vi "Process buy UI.vi"(8 "error in (no error)":errorcluster, 11 "UI Actor in":refnum<class "UI Actor.lvclass">) -> (0 "error out":errorcluster, 3 "UI Actor out":refnum<class "UI Actor.lvclass">)   [LabVIEW 2020, in "UI Actor.lvlib" / "UI Actor.lvclass"]
uses:
  UI Actor.lvclass
  C:/Program Files/National Instruments/LabVIEW 2020/vi.lib/ActorFramework/Actor/Actor.lvclass
  UI Actor.lvclass/UI Actor.ctl
  coffe actor Messages/Productos inventario coffee Msg/Productos inventario coffee Msg.lvclass/Productos inventario coffee Msg.ctl
  <vilib>/ActorFramework/Message Enqueuer/Message Enqueuer.lvclass/Message Enqueuer.ctl
  Soda Actor Messages/Producto inventario Msg/Producto inventario Msg.lvclass/Producto inventario Msg.ctl
  <vilib>/ActorFramework/Actor/Actor.lvclass/Actor.ctl
  MENSAJE Messages/Update MSG Msg/Update MSG Msg.lvclass/Update MSG Msg.ctl
  UI Actor Messages/credit update Msg/credit update Msg.lvclass/credit update Msg.ctl
  <vilib>/ActorFramework/Message Enqueuer/Enqueue.vi
  <vilib>/ActorFramework/Message Enqueuer/Init from Existing Queue.vi
  coffe actor Messages/Productos inventario coffee Msg/Productos inventario coffee Msg.lvclass
  C:/Program Files/National Instruments/LabVIEW 2020/vi.lib/ActorFramework/Message/Message.lvclass
  Soda Actor Messages/Producto inventario Msg/Producto inventario Msg.lvclass
  USD Actor Messages/Credito Reset Msg/Credito Reset Msg.lvclass
  MXN actor Messages/Credito Reset MXN Msg/Credito Reset MXN Msg.lvclass
  MENSAJE Messages/Update MSG Msg/Update MSG Msg.lvclass
  UI Actor Messages/credit update Msg/credit update Msg.lvclass
  <vilib>/Utility/config.llb/Read Key (Double).vi
  <vilib>/ActorFramework/Message Priority Queue/Priority Enqueue.vi
  <vilib>/ActorFramework/Message Enqueuer/Message Enqueuer.lvclass
  <vilib>/Utility/config.llb/NI_LVConfig.lvlib
  <vilib>/ActorFramework/Actor/Actor.lvclass
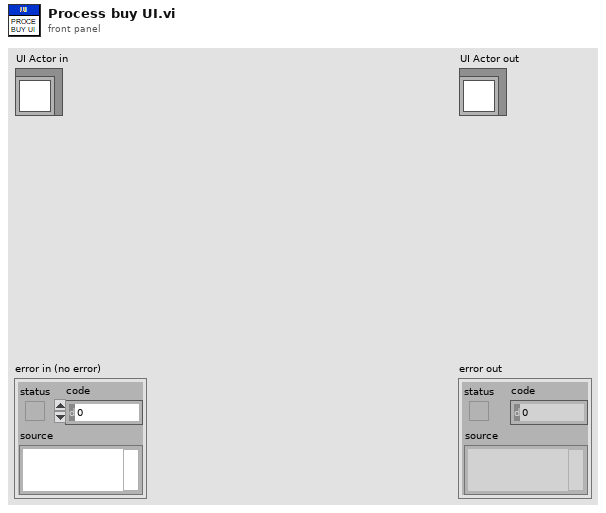
[diagram p1: front panel]
types:
  T1 = typedef "NI_LVConfig.lvlib/Config Data RefNum.ctl" = refnum<k1>
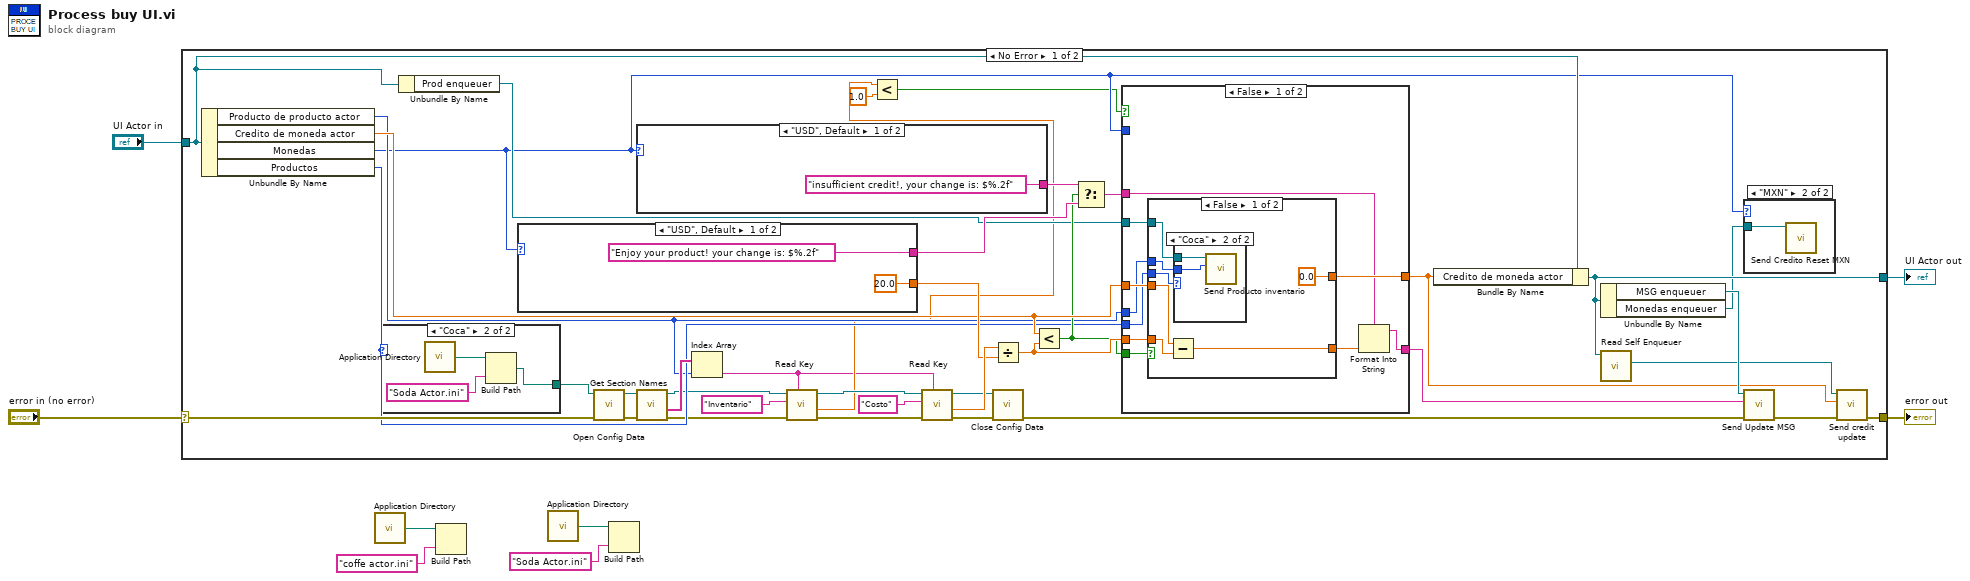
[diagram p0: block diagram]
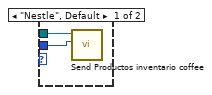
[diagram p2: hidden frame]
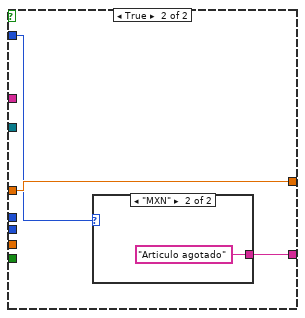
[diagram p4: hidden frame]
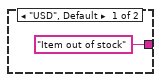
[diagram p5: hidden frame]
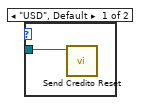
[diagram p6: hidden frame]
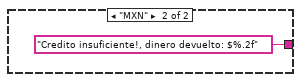
[diagram p7: hidden frame]
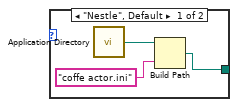
[diagram p8: hidden frame]
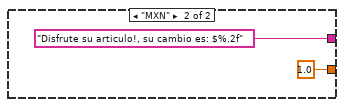
[diagram p9: hidden frame]
diagram:
  n1 = case shown="No Error" "error in (no error)" {
    selector: "error in (no error)" -> [w42 w90]
    tunnel: [w34 w90] -> w7
    tunnel: [w39 w89] -> w5
    tunnel: "UI Actor in" -> [w25 w89]
    frame No Error {
      n2 = Unbundle By Name(w25) -> ("Producto de producto actor"=w23:i32, "Credito de moneda actor"=w31:dbl, "Monedas"=w20:enum16{"USD", "MXN"}, "Productos"=w26:enum16{"Nestle", "Coca"})
      n3 = case shown="\"Coca\"" w26 {
        tunnel: [w79 w82] -> w44
        frame "Nestle", Default {
          n4 = call <vilib>:"Application Directory.vi"() -> ("Application Directory"=w81:path)
          n5 = Build Path(base path=w81, name or relative path="coffe actor.ini") -> (appended path=w79:path)
        }
        frame "Coca" {
          n6 = call <vilib>:"Application Directory.vi"() -> ("Application Directory"=w84:path)
          n7 = Build Path(base path=w84, name or relative path="Soda Actor.ini") -> (appended path=w82:path)
        }
      }
      n8 = Unbundle By Name(w25) -> ("Prod enqueuer"=w24:refnum<class "Message Enqueuer.lvclass">)
      n9 = case shown="\"USD\", Default" w20 {
        tunnel: [20.0 ("y") 1.0 ("y")] -> w40
        tunnel: ["Enjoy your product! your change is: $%.2f" ("format string") "Disfrute su articulo!, su cambio es: $%.2f" ("format string")] -> w33
        frame "USD", Default {
        }
        frame "MXN" {
        }
      }
      n10 = call <vilib>:"Open Config Data.vi"("error in (no error)"=w42, "configuration file path"=w44) -> ("error out"=w47:errorcluster, "refnum"=w46:T1)  [unwired: 7 in, 1 out]
      n11 = case shown="\"USD\", Default" w20 {
        tunnel: ["insufficient credit!, your change is: $%.2f" ("format string") "Credito insuficiente!, dinero devuelto: $%.2f" ("format string")] -> w32
        frame "USD", Default {
        }
        frame "MXN" {
        }
      }
      n12 = call <vilib>:"Get Section Names.vi"("error in (no error)"=w47, "refnum"=w46) -> ("error out"=w19:errorcluster, "section names"=w45:string[], "refnum out"=w13:T1)  [unwired: 7 in]
      n13 = Index Array "Index Array"(array=w45, index=w23) -> (element=w9:string)
      n14 = call-poly <vilib>:"Read Key.vi"("section"=w9, "error in (no error)"=w19, "key"="Inventario", "refnum"=w13) -> ("error out"=w17:errorcluster, "value"=w10:dbl, "refnum out"=w14:T1)  [unwired: 4 in, 1 out]
      n15 = Less?(x=w10, y=1.0) -> (x < y?=w12:bool)
      n16 = call-poly <vilib>:"Read Key.vi"("section"=w9, "error in (no error)"=w17, "key"="Costo", "refnum"=w14) -> ("error out"=w16:errorcluster, "value"=w41:dbl, "refnum out"=w15:T1)  [unwired: 4 in, 1 out]
      n17 = Divide(x=w41, y=w40) -> (x/y=w30:dbl)
      n18 = call <vilib>:"Close Config Data.vi"("error in (no error)"=w16, "refnum"=w15) -> ("error out"=w36:errorcluster)  [unwired: 8 in, 1 out]
      n19 = Less?(x=w31, y=w30) -> (x < y?=w28:bool)
      n20 = Select(t=w32, s=w28, f=w33) -> (s? t:f=w22:string)
      n21 = case shown="False" w12 {
        tunnel: w31 -> [w57 w72]
        tunnel: w30 -> [w56 _]
        tunnel: [w55 w72] -> w29
        tunnel: w28 -> [w54 _]
        tunnel: w26 -> [w53 _]
        tunnel: w24 -> [w52 _]
        tunnel: w23 -> [w51 _]
        tunnel: w22 -> [w49 _]
        tunnel: [w50 w70] -> w21
        tunnel: w20 -> [_ w71]
        frame False {
          n22 = case shown="False" w54 {
            tunnel: w57 -> [w64 w69]
            tunnel: w56 -> [w63 _]
            tunnel: [w62 w69] -> w48
            tunnel: [0.0 ("credito") w69] -> w55
            tunnel: w53 -> [w60 _]
            tunnel: w52 -> [w59 _]
            tunnel: w51 -> [w58 _]
            frame False {
              n23 = Subtract(x=w64, y=w63) -> (x-y=w62:dbl)
              n24 = case shown="\"Coca\"" w60 {
                tunnel: w59 -> [w66 w68]
                tunnel: w58 -> [w65 w67]
                frame "Nestle", Default {
                  n25 = call "Send Productos inventario coffee.vi"("Productos inventario"=w65, "Message Enqueuer"=w66) -> ()  [unwired: 8 in, 2 out]
                }
                frame "Coca" {
                  n26 = call "Send Producto inventario.vi"("Productos inventario"=w67, "Message Enqueuer"=w68) -> ()  [unwired: 8 in, 2 out]
                }
              }
            }
            frame True {
            }
          }
          n27 = Format Into String(format string=w49, w48) -> (resulting string=w50:string)  [unwired: 2 in, 1 out]
        }
        frame True {
          n28 = case shown="\"MXN\"" w71 {
            tunnel: ["Item out of stock" "Articulo agotado"] -> w70
            frame "USD", Default {
            }
            frame "MXN" {
            }
          }
        }
      }
      n29 = Bundle By Name(cluster=w25, "Credito de moneda actor"=w29) -> (w39:refnum<class "UI Actor.lvclass">)
      n30 = Unbundle By Name(w39) -> ("MSG enqueuer"=w38:refnum<class "Message Enqueuer.lvclass">, "Monedas enqueuer"=w27:refnum<class "Message Enqueuer.lvclass">)
      n31 = call <vilib>:"Read Self Enqueuer.vi"("Actor"=w39) -> ("Self Enqueuer"=w37:refnum<class "Message Enqueuer.lvclass">)  [unwired: 10 in]
      n32 = case shown="\"MXN\"" w20 {
        tunnel: w27 -> [w75 w76]
        frame "USD", Default {
          n33 = call "Send Credito Reset.vi"("Message Enqueuer"=w75) -> ()  [unwired: 9 in, 2 out]
        }
        frame "MXN" {
          n34 = call "Send Credito Reset MXN.vi"("Message Enqueuer"=w76) -> ()  [unwired: 9 in, 2 out]
        }
      }
      n35 = call "Send Update MSG.vi"("error in (no error)"=w36, "Update MSG"=w21, "Message Enqueuer"=w38) -> ("error out"=w35:errorcluster)  [unwired: 7 in, 1 out]
      n36 = call "Send credit update.vi"("error in (no error)"=w35, "credito"=w29, "Message Enqueuer"=w37) -> ("error out"=w34:errorcluster)  [unwired: 7 in, 1 out]
    }
    frame Error {
    }
  }
  "error out" <- w7
  "UI Actor out" <- w5
  n37 = call <vilib>:"Application Directory.vi"() -> ("Application Directory"=w3:path)
  n38 = Build Path(base path=w3, name or relative path="coffe actor.ini") -> ()  [unwired: 1 out]
  n39 = call <vilib>:"Application Directory.vi"() -> ("Application Directory"=w1:path)
  n40 = Build Path(base path=w1, name or relative path="Soda Actor.ini") -> ()  [unwired: 1 out]
